vi "I-V扫描脚本.vi"(1 "仪器型号":string, 2 "参数":T1) -> (0 "Script":string)   [LabVIEW 2020]
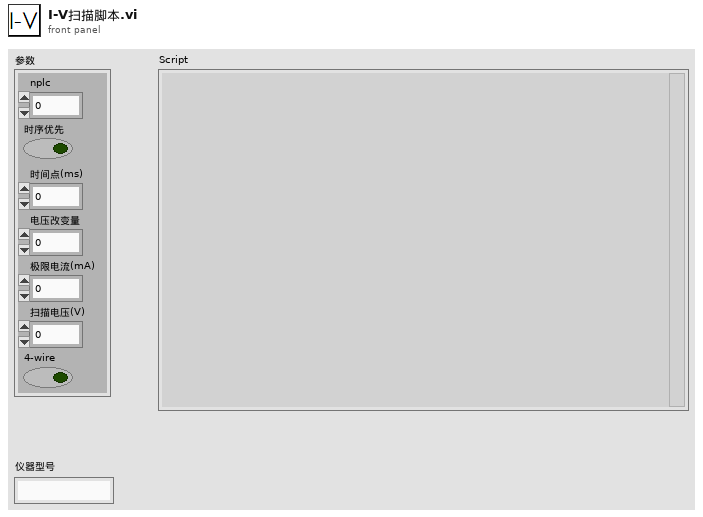
[diagram p1: front panel]
types:
  T1 = cluster{"nplc":dbl, "时序优先":bool, "时间点(ms)":dbl, "电压改变量":dbl, "极限电流(mA)":dbl, "扫描电压(V)":dbl, "4-wire":bool}
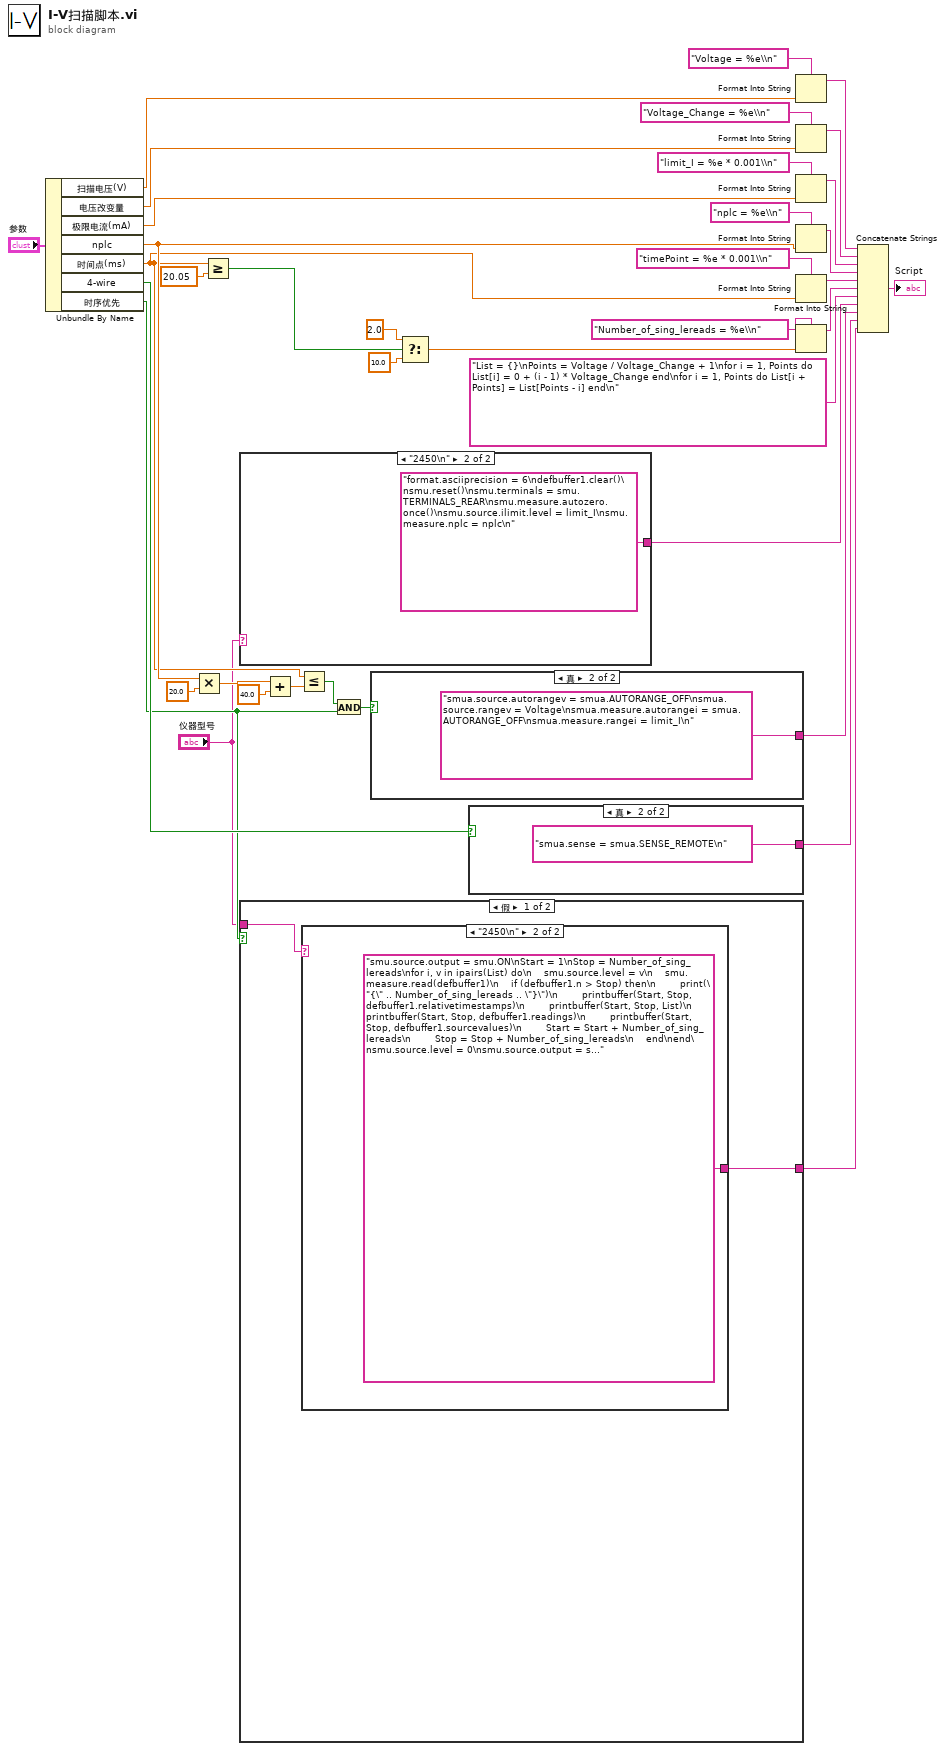
[diagram p0: block diagram]
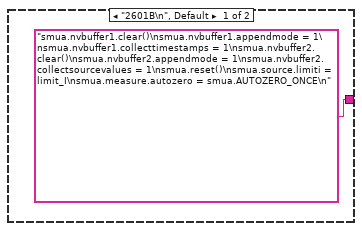
[diagram p2: hidden frame]
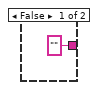
[diagram p3: hidden frame]
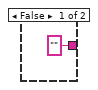
[diagram p4: hidden frame]
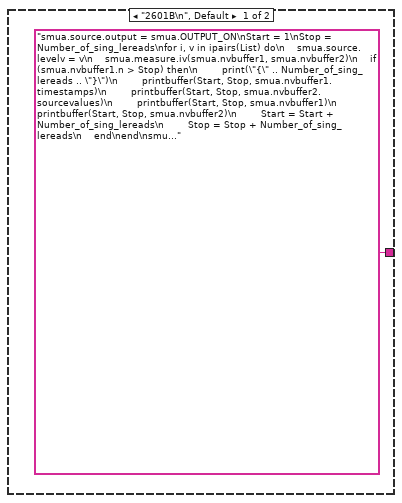
[diagram p5: hidden frame]
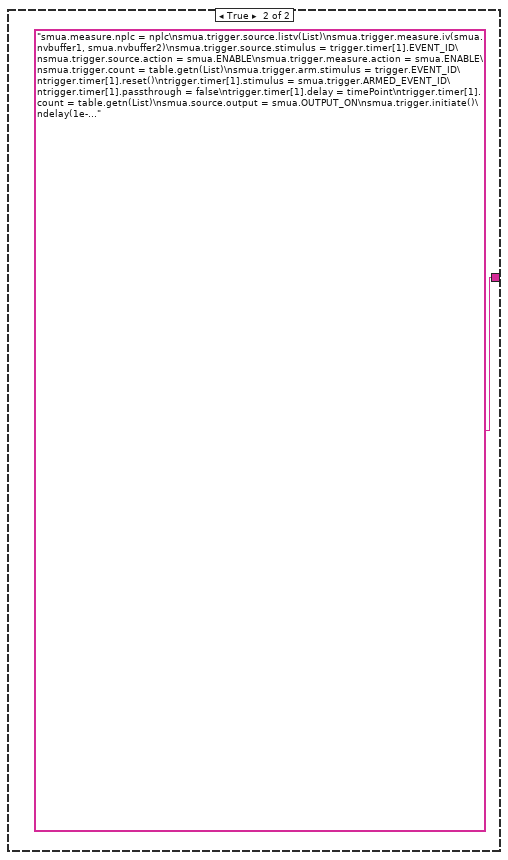
[diagram p6: hidden frame]
diagram:
  n1 = Unbundle By Name("参数") -> ("扫描电压(V)"=w25:dbl, "电压改变量"=w24:dbl, "极限电流(mA)"=w23:dbl, "nplc"=w8:dbl, "时间点(ms)"=w5:dbl, "4-wire"=w22:bool, "时序优先"=w4:bool)
  n2 = Multiply(x=w8, y=20.0) -> (x*y=w11:dbl)
  n3 = Greater Or Equal?(x=w5, y=20.05) -> (x >= y?=w16:bool)
  n4 = case shown="\"2450\\n\"" "仪器型号" {
    tunnel: ["smua.nvbuffer1.clear()\nsmua.nvbuffer1.appendmode = 1\nsmua.nvbuffer1.collecttimestamps = 1\nsmua.nvbuffer2.clear()\nsmua.nvbuffer2.appendmode = 1\nsmua.nvbuffer2.collectsourcevalues = 1\nsmua.reset()\nsmua.source.limiti = limit_I\nsmua.measure.autozero = smua.AUTOZERO_ONCE\n" "format.asciiprecision = 6\ndefbuffer1.clear()\nsmu.reset()\nsmu.terminals = smu.TERMINALS_REAR\nsmu.measure.autozero.once()\nsmu.source.ilimit.level = limit_I\nsmu.measure.nplc = nplc\n"] -> w26
    frame "2601B\n", Default {
    }
    frame "2450\n" {
    }
  }
  n5 = case shown="假" w4 {
    tunnel: [w42 "smua.measure.nplc = nplc\nsmua.trigger.source.listv(List)\nsmua.trigger.measure.iv(smua.nvbuffer1, smua.nvbuffer2)\nsmua.trigger.source.stimulus = trigger.timer[1].EVENT_ID\nsmua.trigger.source.action = smua.ENABLE\nsmua.trigger.measure.action = smua.ENABLE\nsmua.trigger.count = table.getn(List)\nsmua.trigger.arm.stimulus = trigger.EVENT_ID\ntrigger.timer[1].reset()\ntrigger.timer[1].stimulus = smua.trigger.ARMED_EVENT_ID\ntrigger.timer[1].passthrough = false\ntrigger.timer[1].delay = timePoint\ntrigger.timer[1].count = table.getn(List)\nsmua.source.output = smua.OUTPUT_ON\nsmua.trigger.initiate()\ndelay(1e-3)\nsmua.trigger.arm.set()\nfunction _done()\n    Start = 1\n    Stop = Number_of_sing_lereads\n    repeat\n        if (bit.test(status.operation.instrument.smua.condition, 4) == false) then\n            smua.source.leveli = 0\n            smua.source.levelv = 0\n            smua.source.output = smua.OUTPUT_OFF\n            Stop = table.getn(List)\n            print(\"{\" .. Stop - Start + 1 .. \"}\")\n            printbuffer(Start, Stop, smua.nvbuffer1.timestamps)\n            printbuffer(Start, Stop, smua.nvbuffer2.sourcevalues)\n            printbuffer(Start, Stop, smua.nvbuffer1)\n            printbuffer(Start, Stop, smua.nvbuffer2)\n            print(\"{done}\")\n            return\n        elseif (smua.nvbuffer1.n > Stop) then\n            print(\"{\" .. Number_of_sing_lereads .. \"}\")\n            printbuffer(Start, Stop, smua.nvbuffer1.timestamps)\n            printbuffer(Start, Stop, smua.nvbuffer2.sourcevalues)\n            printbuffer(Start, Stop, smua.nvbuffer1)\n            printbuffer(Start, Stop, smua.nvbuffer2)\n            Start = Start + Number_of_sing_lereads\n            Stop = Stop + Number_of_sing_lereads\n        end\n        delay(timePoint)\n    until (false)\nend\n_done()\nreset()"] -> w21
    tunnel: "仪器型号" -> [w41 _]
    frame False {
      n6 = case shown="\"2450\\n\"" w41 {
        tunnel: ["smua.source.output = smua.OUTPUT_ON\nStart = 1\nStop = Number_of_sing_lereads\nfor i, v in ipairs(List) do\n    smua.source.levelv = v\n    smua.measure.iv(smua.nvbuffer1, smua.nvbuffer2)\n    if (smua.nvbuffer1.n > Stop) then\n        print(\"{\" .. Number_of_sing_lereads .. \"}\")\n        printbuffer(Start, Stop, smua.nvbuffer1.timestamps)\n        printbuffer(Start, Stop, smua.nvbuffer2.sourcevalues)\n        printbuffer(Start, Stop, smua.nvbuffer1)\n        printbuffer(Start, Stop, smua.nvbuffer2)\n        Start = Start + Number_of_sing_lereads\n        Stop = Stop + Number_of_sing_lereads\n    end\nend\nsmua.source.levelv = 0\nsmua.source.uotput = smua.OUTPUT_OFF\nStop = table.getn(List)\nprint(\"{\" .. Stop - Start + 1 .. \"}\")\nprintbuffer(Start, Stop, smua.nvbuffer1.timestamps)\nprintbuffer(Start, Stop, smua.nvbuffer2.sourcevalues)\nprintbuffer(Start, Stop, smua.nvbuffer1)\nprintbuffer(Start, Stop, smua.nvbuffer2)\nprint(\"{done}\")\nreset()" "smu.source.output = smu.ON\nStart = 1\nStop = Number_of_sing_lereads\nfor i, v in ipairs(List) do\n    smu.source.level = v\n    smu.measure.read(defbuffer1)\n    if (defbuffer1.n > Stop) then\n        print(\"{\" .. Number_of_sing_lereads .. \"}\")\n        printbuffer(Start, Stop, defbuffer1.relativetimestamps)\n        printbuffer(Start, Stop, List)\n        printbuffer(Start, Stop, defbuffer1.readings)\n        printbuffer(Start, Stop, defbuffer1.sourcevalues)\n        Start = Start + Number_of_sing_lereads\n        Stop = Stop + Number_of_sing_lereads\n    end\nend\nsmu.source.level = 0\nsmu.source.output = smu.OFF\nStop = table.getn(List)\nprint(\"{\" .. Stop - Start + 1 .. \"}\")\nprintbuffer(Start, Stop, defbuffer1.relativetimestamps)\nprintbuffer(Start, Stop, List)\nprintbuffer(Start, Stop, defbuffer1.readings)\nprintbuffer(Start, Stop, defbuffer1.sourcevalues)\nprint(\"{done}\")"] -> w42
        frame "2601B\n", Default {
        }
        frame "2450\n" {
        }
      }
    }
    frame True {
    }
  }
  n7 = Add(x=w11, y=40.0) -> (x+y=w9:dbl)
  n8 = Less Or Equal?(x=w5, y=w9) -> (x <= y?=w3:bool)
  n9 = And(x=w3, y=w4) -> (x .and. y?=w2:bool)
  n10 = case shown="真" w2 {
    tunnel: ["" "smua.source.autorangev = smua.AUTORANGE_OFF\nsmua.source.rangev = Voltage\nsmua.measure.autorangei = smua.AUTORANGE_OFF\nsmua.measure.rangei = limit_I\n"] -> w7
    frame False {
    }
    frame True {
    }
  }
  n11 = Select(t=2.0, s=w16, f=10.0) -> (s? t:f=w13:dbl)
  n12 = case shown="真" w22 {
    tunnel: ["" "smua.sense = smua.SENSE_REMOTE\n"] -> w6
    frame False {
    }
    frame True {
    }
  }
  n13 = Format Into String(format string="Voltage = %e\\n" ("格式字符串"), w25) -> (resulting string=w35:string)  [unwired: 2 in, 1 out]
  n14 = Format Into String(format string="Voltage_Change = %e\\n" ("格式字符串"), w24) -> (resulting string=w33:string)  [unwired: 2 in, 1 out]
  n15 = Format Into String(format string="limit_I = %e * 0.001\\n" ("格式字符串"), w23) -> (resulting string=w32:string)  [unwired: 2 in, 1 out]
  n16 = Format Into String(format string="nplc = %e\\n", w8) -> (resulting string=w30:string)  [unwired: 2 in, 1 out]
  n17 = Format Into String(format string="timePoint = %e * 0.001\\n", w5) -> (resulting string=w28:string)  [unwired: 2 in, 1 out]
  n18 = Format Into String(format string="Number_of_sing_lereads = %e\\n" ("格式字符串"), w13) -> (resulting string=w19:string)  [unwired: 2 in, 1 out]
  n19 = Concatenate Strings(w35, w33, w32, w30, w28, w19, "List = {}\nPoints = Voltage / Voltage_Change + 1\nfor i = 1, Points do List[i] = 0 + (i - 1) * Voltage_Change end\nfor i = 1, Points do List[i + Points] = List[Points - i] end\n", w26, w7, w6, w21) -> (→"Script":string)
